vi "Node Controller Initialize.vi"(8 "error in (no error)":errorcluster, 11 "Simple Map Node Controller in":refnum<class "Simple Numeric Map Node Controller.lvclass">) -> (0 "error out":errorcluster, 3 "Simple Map Node Controller out":refnum<class "Simple Numeric Map Node Controller.lvclass">)   [LabVIEW 2024, in "Simple Numeric Map Node Controller.lvclass"]
uses:
  Simple Numeric Map Node Controller.lvclass
  Simple Numeric Map Node Controller.lvclass/Simple Numeric Map Node Controller.ctl
  Ancestor Class/Messenger/Mail Strategy/Mail Strategy.lvclass
  Ancestor Class/Actor/System Actor/System Actor.lvclass
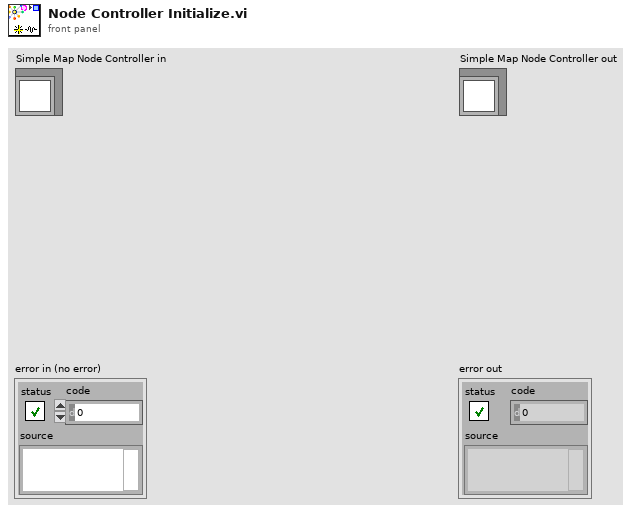
[diagram p1: front panel]
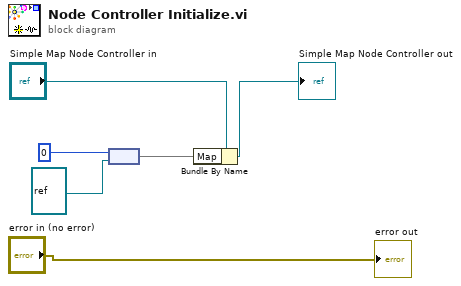
[diagram p0: block diagram]
diagram:
  n1 = node(i64 0, refnum<vi> refnum ("Node VI Ref")) -> (w3:map{i64, refnum<vi>})
  n2 = Bundle By Name(cluster="Simple Map Node Controller in", "Map"=w3) -> (→"Simple Map Node Controller out":refnum<class "Simple Numeric Map Node Controller.lvclass">)
  "error out" <- "error in (no error)"
